vi "test_Path (appdir).vi"(8 "error in (no error)":errorcluster, 11 "TestCase in":refnum<class "Read Section - Path Tests.lvclass">) -> (0 "error out":errorcluster, 3 "TestCase out":refnum<class "Read Section - Path Tests.lvclass">)   [LabVIEW 2017, in "Read Section - Path Tests.lvclass"]
uses:
  Read Section - Path Tests.lvclass
  C:/Development/Reuse-libraries/File IO/_Unit Test/Read File Tests/Read File Tests.lvclass
  Read File Tests.lvclass/Read File Tests.ctl
  Read/Read Section - Path.vi
  <vilib>/addons/_JKI Toolkits/VI Tester/TestCase.llb/TestCase.lvclass
  TSC File IO.lvlib
  Read File Tests.lvclass
  C:/Program Files (x86)/National Instruments/LabVIEW 2017/vi.lib/addons/_JKI Toolkits/VI Tester/TestCase.llb/TestCase.lvclass
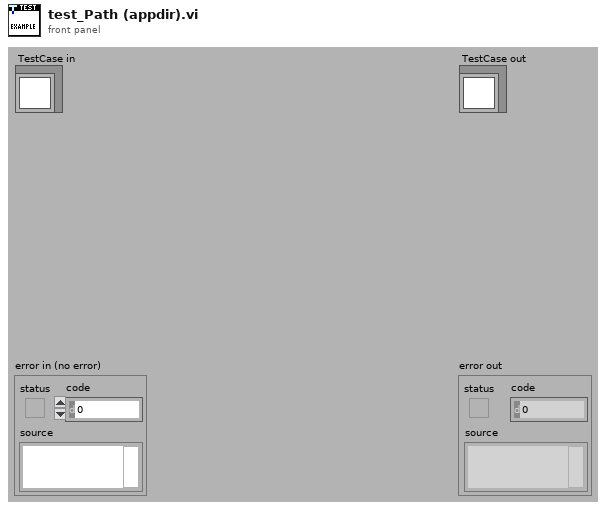
[diagram p1: front panel]
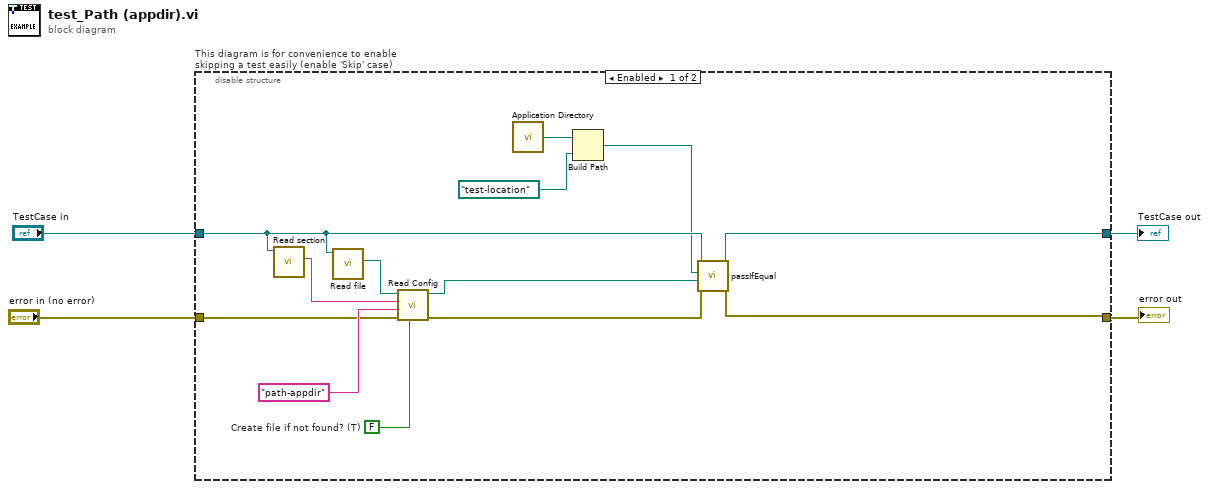
[diagram p0: block diagram]
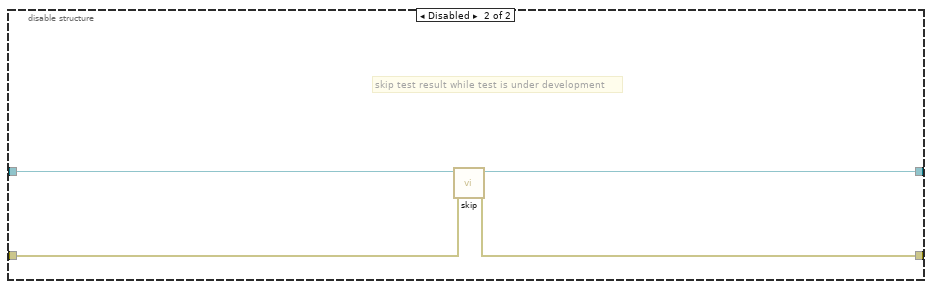
[diagram p2: hidden frame]
diagram:
  n1 = disable-structure "This diagram is for convenience to enable skipping a test easily (enable 'Skip' case)" shown="Enabled" {
    disable-tunnel: "TestCase in" -> [w10 w21]
    disable-tunnel: [w17 w19] -> w1
    disable-tunnel: [w16 w20] -> w3
    disable-tunnel: "error in (no error)" -> [w13 w18]
    frame Enabled {
      w14 = FALSE  # Create file if not found? (T)
      n2 = call "Read section.vi"("Read File Tests in"=w10) -> ("section"=w9:string)  [unwired: 8 in, 2 out]
      n3 = call "Read file.vi"("Read File Tests in"=w10) -> ("file"=w11:path)  [unwired: 8 in, 2 out]
      n4 = call-poly "Read Config.vi"("Create file if not found? (T)"=w14, "error in (no error)"=w13, "key"="path-appdir", "section"=w9, "Path"=w11) -> ("error out"=w12:errorcluster, "value"=w8:path)  [unwired: 5 in]
      n5 = call <vilib>:"Application Directory.vi"() -> ("Application Directory"=w7:path)
      n6 = Build Path(base path=w7, name or relative path=path "test-location") -> (appended path=w5:path)
      n7 = call-dynamic "passIfEqual.vi"("error in (no error)"=w12, "y"=w8, "x"=w5, "TestCase in"=w10) -> ("error out"=w16:errorcluster, "TestCase out"=w17:refnum<class "Read Section - Path Tests.lvclass">)  [unwired: 6 in]
    }
    frame Disabled {
      # "skip test result while test is under development"
      n8 = call <vilib>:"skip.vi"("error in (no error)"=w18, "TestCase in"=w21) -> ("error out"=w20:errorcluster, "TestCase out"=w19:refnum<class "Read Section - Path Tests.lvclass">)  [unwired: 8 in]
    }
  }
  "error out" <- w3
  "TestCase out" <- w1
